vi "PH_Beckhoff_PP_PU.read DB.vi"(3 "error in":errorcluster, 5 "Instance Name":string) -> (0 "error out":errorcluster, 1 "PSU Info":T2, 2 "HV Meas Info":T1)   [LabVIEW 2014, in "PH_Beckhoff_PP_PU.lvlib"]
doc: "This VI reads information from the database."
uses:
  PH_Beckhoff_PP_PU.lvlib
  PH_Beckhoff_PP_PU.PSU Info.ctl
  PH_Beckhoff_PP_PU.HV Meas Info.ctl
  PH_Common/PH_Common.lvlib
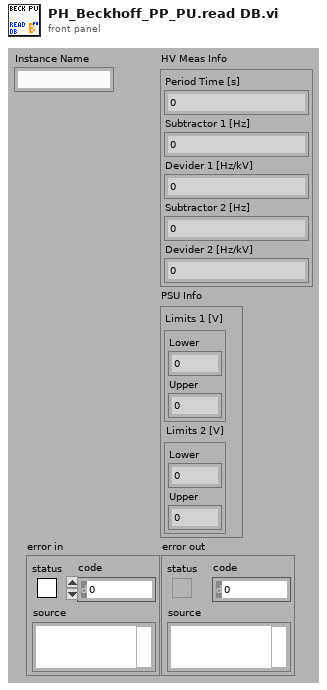
[diagram p1: front panel]
types:
  T1 = typedef "PH_Beckhoff_PP_PU.lvlib/PH_Beckhoff_PP_PU.HV Meas Info.ctl" = cluster{"Period Time [s]":dbl, "Subtractor 1 [Hz]":dbl, "Devider 1 [Hz/kV]":dbl, "Subtractor 2 [Hz]":dbl, "Devider 2 [Hz/kV]":dbl}
  T2 = typedef "PH_Beckhoff_PP_PU.lvlib/PH_Beckhoff_PP_PU.PSU Info.ctl" = cluster{"Limits 1 [V]":cluster{"Lower":dbl, "Upper":dbl}, "Limits 2 [V]":cluster{"Lower":dbl, "Upper":dbl}}
  T3 = cluster{"[0]":dbl, "[1]":dbl, "[2]":dbl, "[3]":dbl, "[4]":dbl}
  T4 = cluster{cluster{"[0]":dbl, "[1]":dbl}, cluster{"[0]":dbl, "[1]":dbl}}
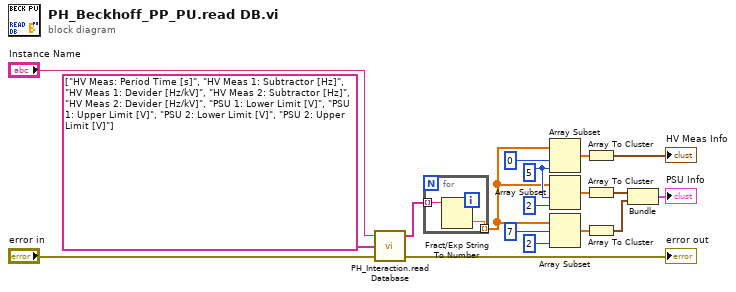
[diagram p0: block diagram]
diagram:
  w9 = 5 ("index")
  n1 = call "PH_Interaction.read Database.vi"("error in (no error)"="error in", "Strings to search for"=string[] ["HV Meas: Period Time [s]", "HV Meas 1: Subtractor [Hz]", "HV Meas 1: Devider [Hz/kV]", "HV Meas 2: Subtractor [Hz]", "HV Meas 2: Devider [Hz/kV]", "PSU 1: Lower Limit [V]", "PSU 1: Upper Limit [V]", "PSU 2: Lower Limit [V]", "PSU 2: Upper Limit [V]"] ("Strings to search for in"), "DB Entry to read"="Instance Name") -> ("error out"=→"error out":errorcluster, "Values"=w13:string[])  [unwired: 1 in]
  n2 = for {
    tunnel: w13 -> [w20] mode=indexing
    tunnel: [w19] -> w3 mode=indexing
    n3 = Fract/Exp String To Number(string=w20) -> (number=w19:dbl)  [unwired: 3 in, 1 out]
  }
  n4 = Array Subset(array=w3, index=0 ("length"), length=w9) -> (w11:dbl[])
  n5 = Array Subset(array=w3, index=w9, length=2) -> (w7:dbl[])
  n6 = Array Subset(array=w3, index=7, length=2) -> (w2:dbl[])
  n7 = Array To Cluster(array=w11) -> (cluster=→"HV Meas Info":T3)
  n8 = Array To Cluster(array=w7) -> (cluster=w6:cluster{"[0]":dbl, "[1]":dbl})
  n9 = Array To Cluster(array=w2) -> (cluster=w1:cluster{"[0]":dbl, "[1]":dbl})
  n10 = Bundle(w6, w1) -> (→"PSU Info":T4)  [unwired: 1 in]
